vi "State Machin test.vi"(11 "Array":dbl[](array[numeric])) -> (3 "Numeric":dbl)   [LabVIEW 2019]
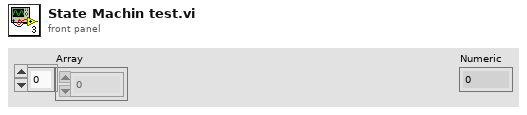
[diagram p1: front panel]
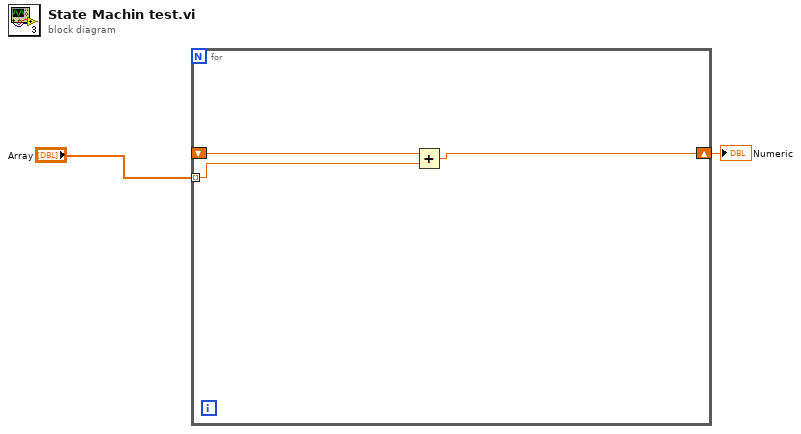
[diagram p0: block diagram]
diagram:
  n1 = for {
    tunnel: "Array" -> [w5] mode=indexing
    shift-right: [w4] -> w1
    shift-left: _ -> [w3]
    n2 = Add(x=w3, y=w5) -> (x+y=w4:dbl)
  }
  "Numeric" <- w1
